vi "Pre Launch Init.vi"(11 "Controller in":refnum<class "Controller.lvclass">) -> (0 "error out":errorcluster, 3 "Controller out":refnum<class "Controller.lvclass">)   [LabVIEW 2016, in "Controller.lvlib" / "Controller.lvclass"]
doc: "(<B>Filename</B>: Actor Framework.lvlib:Actor.lvclass:Pre Launch Init.vi)\n\nDefines behavior that occurs after the Launch Nested Actor method is invoked but before the actor's Actor Core method begins running.\n\nBy default, this method does nothing. A descendant class may override it to define behavior."
uses:
  Controller.lvclass
  UI/UI/Controls/Start Acquisition.ctl
  <vilib>/userdefined/High Color/IMAQdx.ctl
  Controller.lvclass/Controller.ctl
  <vilib>/ActorFramework/Actor/Actor.lvclass
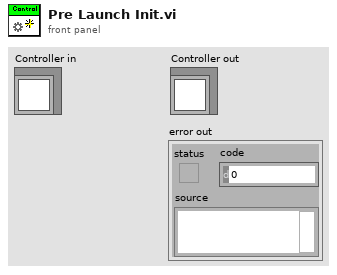
[diagram p1: front panel]
types:
  T1 = typedef "Start Acquisition.ctl" = cluster{"Image Indicator Reference":refnum<vi>, "Start":bool, "Camera":T2}
  T2 = typedef "IMAQdx.ctl" = refnum<k21>
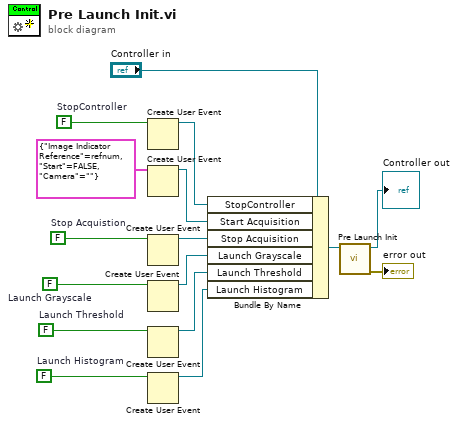
[diagram p0: block diagram]
diagram:
  w4 = FALSE  # Launch Histogram
  w5 = FALSE  # Launch Threshold
  w6 = FALSE  # Launch Grayscale
  w10 = FALSE  # Stop Acquistion
  w14 = FALSE  # StopController
  n1 = Create User Event(user event datatype=w14) -> (user event=w13:refnum<user-event>)  [unwired: 1 in, 1 out]
  n2 = Create User Event(user event datatype=T1 {"Image Indicator Reference"=refnum, "Start"=FALSE, "Camera"=""} ("Start Acquisition")) -> (user event=w7:refnum<user-event>)  [unwired: 1 in, 1 out]
  n3 = Create User Event(user event datatype=w10) -> (user event=w9:refnum<user-event>)  [unwired: 1 in, 1 out]
  n4 = Create User Event(user event datatype=w6) -> (user event=w3:refnum<user-event>)  [unwired: 1 in, 1 out]
  n5 = Create User Event(user event datatype=w5) -> (user event=w2:refnum<user-event>)  [unwired: 1 in, 1 out]
  n6 = Create User Event(user event datatype=w4) -> (user event=w1:refnum<user-event>)  [unwired: 1 in, 1 out]
  n7 = Bundle By Name(cluster="Controller in", "StopController"=w13, "Start Acquisition"=w7, "Stop Acquisition"=w9, "Launch Grayscale"=w3, "Launch Threshold"=w2, "Launch Histogram"=w1) -> (w11:refnum<class "Controller.lvclass">)
  n8 = call-parent "Pre Launch Init.vi"("Actor in"=w11) -> ("error out"=→"error out":errorcluster, "Actor out"=→"Controller out":refnum<class "Controller.lvclass">)  [unwired: 9 in]
